vi "Display Console - Show Transaction.vi"(8 "error in (no error)":errorcluster, 11 "Transactions":T1) -> (0 "error out":errorcluster, 3 "Transaction Name":string)   [LabVIEW 2017]
doc: "Translates current active transaction from TypeDef to STR message for displaying Transaction name."
uses:
  User Console View/Controls/User Console - Transactions.ctl
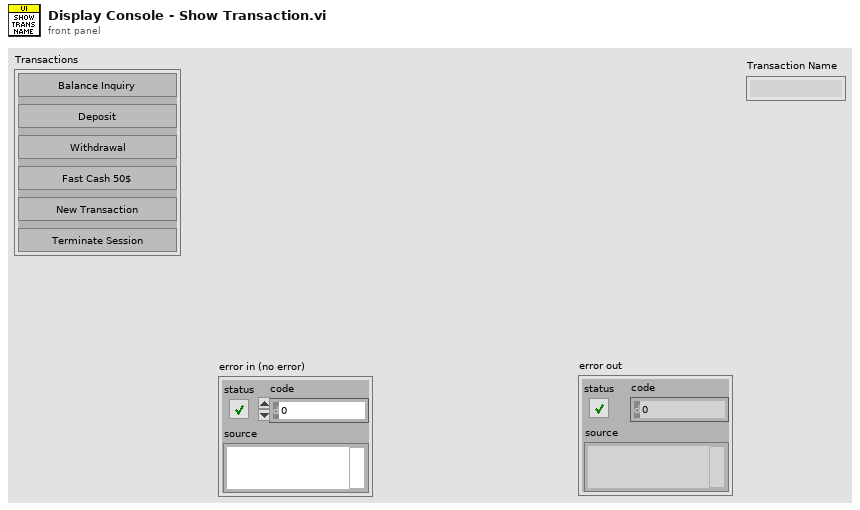
[diagram p1: front panel]
types:
  T1 = typedef "User Console - Transactions.ctl" = cluster{"Balance Inquiry":bool, "Deposit":bool, "Withdrawal":bool, "Fast Cash":bool, "New Transaction":bool, "Terminate":bool}
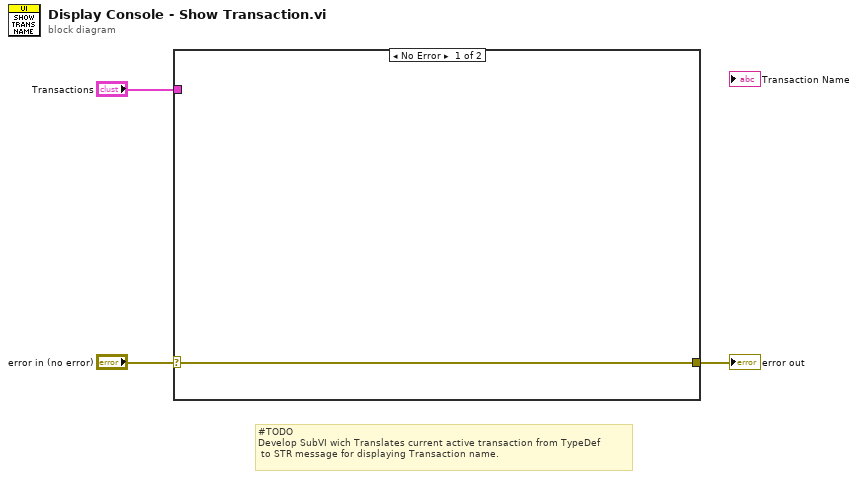
[diagram p0: block diagram]
diagram:
  # "#TODO\nDevelop SubVI wich Translates current active transaction from TypeDef\n to STR message for displaying Transaction name."
  n1 = case shown="No Error" "error in (no error)" {
    selector: "error in (no error)" -> [w4 _]
    tunnel: [w4 _] -> w2
    tunnel: "Transactions" -> [_ _]
    frame No Error {
    }
    frame Error {
    }
  }
  "error out" <- w2
